vi "Read SEQ.vi"(9 "SEQ file path":path, 10 "Sequence files handle":T1) -> (0 "error out":errorcluster, 1 "AOI List":i16[][](array[numeric]), 2 "# of Frames":i16)   [LabVIEW 2011]
uses:
  Sequence files handle.ctt
  GLIMPSE Globals.vi
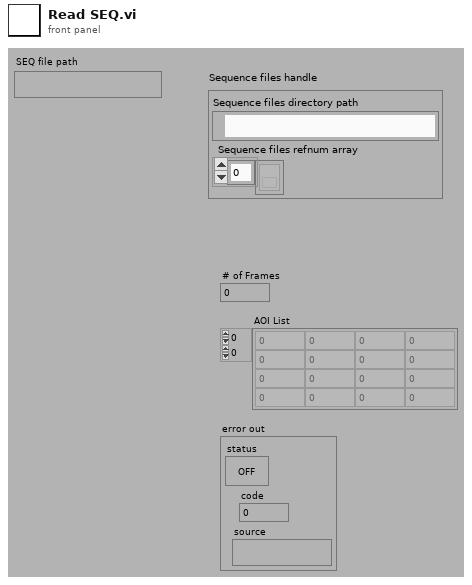
[diagram p1: front panel]
types:
  T1 = typedef "Sequence files handle.ctt" = cluster{"Sequence files directory path":path, "Sequence files refnum array":refnum<file>[]}
  T2 = enum32{"existing file", "new file", "new or existing file", "existing dir", "new dir", "new or existing dir", "existing file (use LLBs)", "new file (use LLBs)", "new or existing file (use LLBs)", "new or existing file or directory (use LLBs)"}
  T3 = cluster{"second":i32, "minute":i32, "hour":i32, "day of month":i32, "month":i32, "year":i32, "day of week":i32, "day of year":i32, "is DST":i32}
  T4 = cluster{"User Name":string, "Description":string, "Time Info":string}
  T5 = typedef "Offset table.ctl" = cluster{"offset":T6, "file number":T7}[]
  T6 = typedef "Offset.ctl" = i32
  T7 = typedef "file number.ctl" = u8
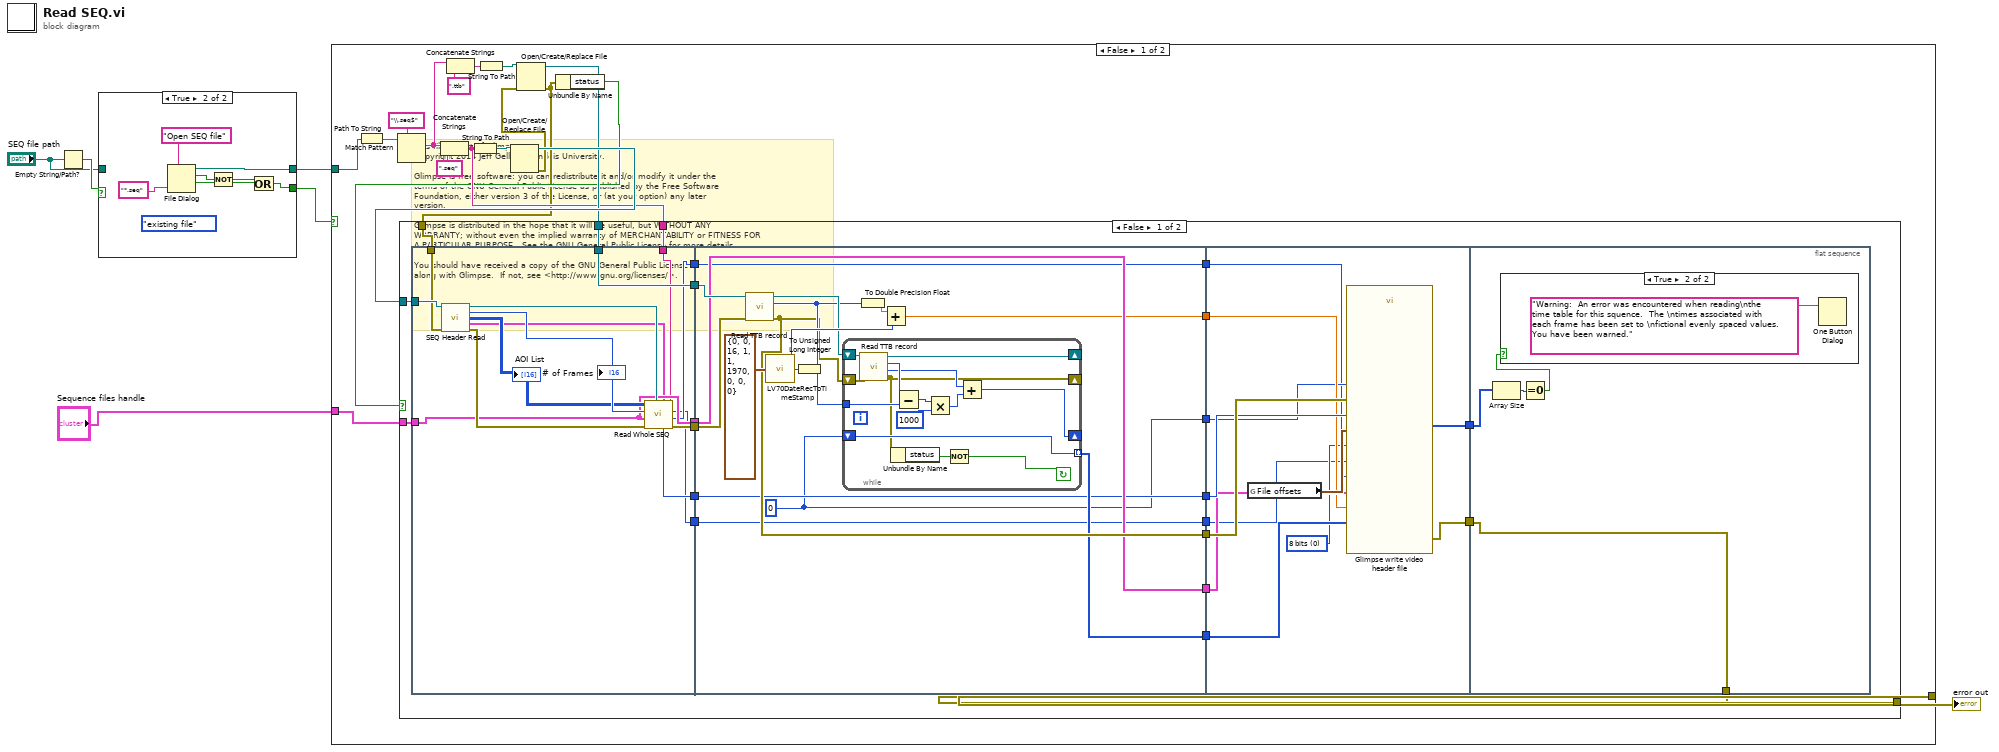
[diagram p0: block diagram]
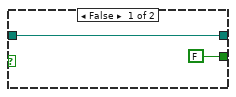
[diagram p2: hidden frame]
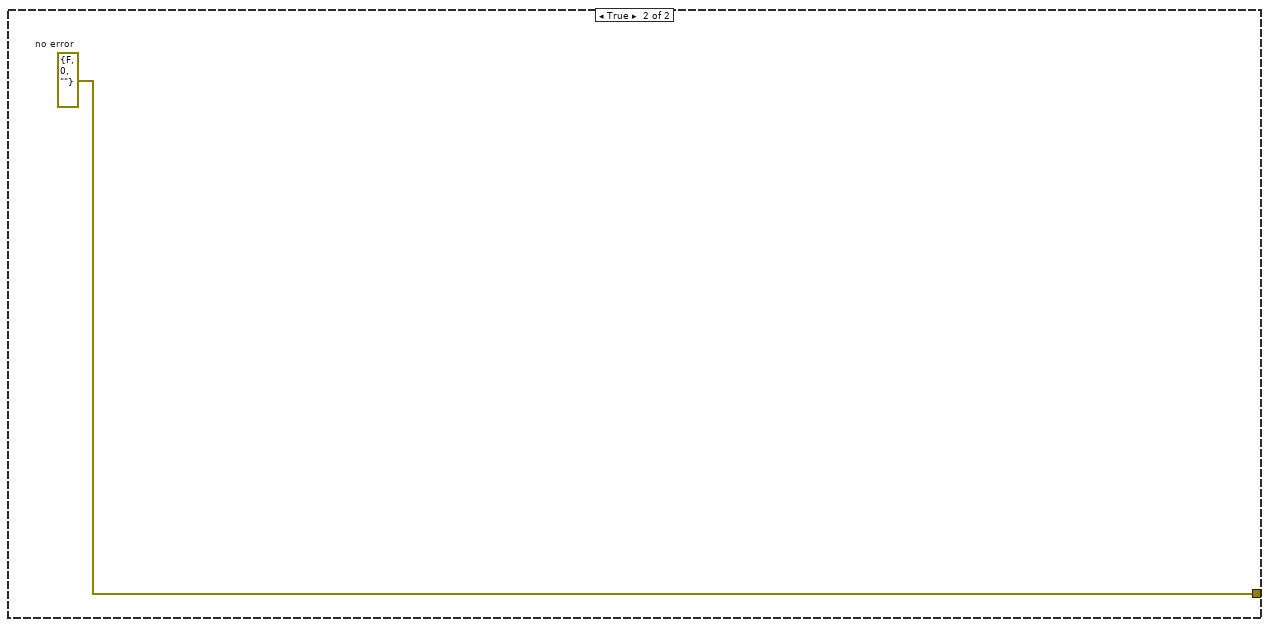
[diagram p5: hidden frame]
diagram:
  # "This file is part of Glimpse. \nCopyright 2014 Jeff Gelles, Brandeis University.    \n\nGlimpse is free software: you can redistribute it and/or modify it under the \nterms of the GNU General Public License as published by the Free Software \nFoundation, either version 3 of the License, or (at your option) any later \nversion.\n\nGlimpse is distributed in the hope that it will be useful, but WITHOUT ANY \nWARRANTY; without even the implied warranty of MERCHANTABILITY or FITNESS FOR \nA PARTICULAR PURPOSE.  See the GNU General Public License for more details.\n\nYou should have received a copy of the GNU General Public License\nalong with Glimpse.  If not, see <http://www.gnu.org/licenses/>."
  n1 = Empty String/Path?(string/path="SEQ file path") -> (empty?=w6:bool)
  n2 = case shown="True" w6 {
    tunnel: [w8 w15] -> w3
    tunnel: "SEQ file path" -> [w8 _]
    tunnel: [FALSE ("cancelled") w11] -> w4
    frame False {
    }
    frame True {
      (unwired) T2."existing file" ("select mode (2)")
      n3 = File Dialog(6:"*.seq" ("pattern"), 7:"Open SEQ file" ("prompt")) -> (1:w12:bool, 2:w14:bool, 3:w15:path)  [unwired: 1 in, 5 out]
      n4 = Not(x=w14) -> (.not. x?=w13:bool)
      n5 = Or(x=w13, y=w12) -> (x .or. y?=w11:bool)
    }
  }
  n6 = case shown="False" w4 {
    tunnel: [w17 w116] -> w2
    tunnel: w3 -> [w30 _]
    tunnel: "Sequence files handle" -> [w16 _]
    frame False {
      n7 = Path To String(path=w30) -> (string=w29:string)
      n8 = Match Pattern(string=w29, regular expression="\\.seq$") -> (before substring=w23:string)  [unwired: 4 out]
      n9 = Concatenate Strings(w23, ".seq") -> (w21:string)
      n10 = Concatenate Strings(w23, ".ttb") -> (w25:string)
      n11 = String To Path(string=w21) -> (path=w28:path)
      n12 = String To Path(string=w25) -> (path=w26:path)
      n13 = Open/Create/Replace File(file path (use dialog)=w28) -> (refnum out=w27:refnum<file>, error out=w20:errorcluster)  [unwired: 1 in, 5 out]
      n14 = Open/Create/Replace File(file path (use dialog)=w26, error in=w20) -> (refnum out=w22:refnum<file>, error out=w18:errorcluster)  [unwired: 5 out]
      n15 = Unbundle By Name(w18) -> ("status"=w19:bool)
      n16 = case shown="False" w19 {
        tunnel: [w50 w115] -> w17
        tunnel: w27 -> [w54 _]
        tunnel: w22 -> [w53 _]
        tunnel: w21 -> [w52 _]
        tunnel: w18 -> [w37 w115]
        tunnel: w16 -> [w51 _]
        frame False {
          n17 = flat-sequence {
            tunnel: w54 -> [w68]
            tunnel: w53 -> [w60]
            tunnel: [w60] -> w49
            tunnel: w52 -> [w59]
            tunnel: w51 -> [w62]
            tunnel: [w62] -> w48
            tunnel: [w63] -> w47
            tunnel: [w61] -> w46
            tunnel: w37 -> [w57]
            tunnel: [w56] -> w35
            tunnel: [w55] -> w33
            tunnel: w49 -> [w84]
            tunnel: w48 -> [w74]
            tunnel: [w74] -> w45
            tunnel: w47 -> [w83]
            tunnel: [w76] -> w44
            tunnel: [w77] -> w43
            tunnel: w46 -> [w73]
            tunnel: [w73] -> w42
            tunnel: [w72] -> w39
            tunnel: [w71] -> w38
            tunnel: [w70] -> w36
            tunnel: w35 -> [w70]
            tunnel: [w69] -> w34
            tunnel: w33 -> [w69]
            tunnel: w45 -> [w104]
            tunnel: [w105] -> w41
            tunnel: w44 -> [w109]
            tunnel: [w109] -> w40
            tunnel: w43 -> [w108]
            tunnel: w42 -> [w106]
            tunnel: w39 -> [w103]
            tunnel: w38 -> [w102]
            tunnel: w36 -> [w100]
            tunnel: w34 -> [w99]
            tunnel: [w110] -> w50
            tunnel: w41 -> [w110]
            tunnel: w40 -> [w112]
            frame #0 {
              n18 = call "SEQ Header Read.vi"("refnum"=w68, "error in"=w57) -> ("refnum out"=w67:refnum<file>, "# of Frames"=w66:i16, "AOI List"=w65:i16[][], "Header Info"=w58:T4, "error out"=w64:errorcluster)  [unwired: 1 in, 8 out]
              "# of Frames" <- w66
              "AOI List" <- w65
              n19 = call "Read Whole SEQ.vi"("AOI List"=w65, "# of Frames"=w66, "Output Sequence files handle"=w62, "error in"=w64, "SEQ file refnum"=w67, "Header Info"=w58, "File name"=w59) -> ("# of frames read"=w61:i32, "Frame height"=w55:i16, "Frame width"=w56:i16, "error out"=w63:errorcluster)
            }
            frame #1 {
              w71 = u32 0 ("Element 0 of TTB")
              n20 = call "Read TTB record.vi"("error in"=w83, "Refnum"=w84) -> ("error out"=w77:errorcluster, "seconds"=w78:u32, "Duplicate Refnum"=w79:refnum<file>)  [unwired: 7 out]
              n21 = call <vilib>:"LV70DateRecToTimeStamp.vi"("date time rec"=T3 {"second"=0, "minute"=0, "hour"=16, "day of month"=1, "month"=1, "year"=1970, "day of week"=0, "day of year"=0, "is DST"=0}) -> ("Time Stamp"=w75:timestamp)
              n22 = To Unsigned Long Integer(number=w75) -> (unsigned 32bit integer=w80:u32)
              n23 = while {
                shift-right: [w96] -> _
                shift-left: w79 -> [w97]
                shift-right: [w87] -> _
                shift-left: w77 -> [w98]
                tunnel: w78 -> [w94]
                shift-right: [w89] -> _
                shift-left: w71 -> [w88]
                tunnel: [w88] -> w76 mode=indexing
                stop <- w85 continue-if-true
                n24 = call "Read TTB record.vi"("error in"=w98, "Refnum"=w97) -> ("error out"=w87:errorcluster, "milliseconds"=w91:u16, "seconds"=w95:u32, "Duplicate Refnum"=w96:refnum<file>)  [unwired: 6 out]
                n25 = Unbundle By Name(w87) -> ("status"=w86:bool)
                n26 = Subtract(x=w95, y=w94) -> (x-y=w93:u32)
                n27 = Multiply(x=w93, y=u32 1000) -> (x*y=w92:u32)
                n28 = Not(x=w86) -> (.not. x?=w85:bool)
                n29 = Add(x=w91, y=w92) -> (x+y=w89:u32)
              }
              n30 = To Double Precision Float(number=w78) -> (double precision float=w81:dbl)
              n31 = Add(x=w81, y=w80) -> (x+y=w72:dbl)
            }
            frame #2 {
              w101 = u32 0 items=["8 bits", "16 bits", "Float", "Complex", "RGB", "HSL"] ("Current sequence pixel depth\n(0=8 bit; 1= 16 bit)")
              n32 = global read "GLIMPSE Globals.vi" "File offsets"() -> (w107:T5)
              n33 = call "Glimpse write video header file.vi"("Number of frames"=w106, "Sequence files handle"=w104, "Pixel depth\n(0=8 bit; 1= 16 bit)"=w101, "error in"=w108, "TTB Array"=w109, "Offsets Array"=w107, "Region width"=w100, "Region height"=w99, "Element 0 of TTB"=w102, "time of 1st frame, \nsec since 1/1/04"=w103) -> ("error out"=w105:errorcluster)  [unwired: 9 in]
            }
            frame #3 {
              n34 = Array Size(array=w112) -> (size(s)=w113:i32)
              n35 = Equal To 0?(x=w113) -> (x = 0?=w111:bool)
              n36 = case shown="True" w111 {
                frame False {
                }
                frame True {
                  n37 = One Button Dialog(message="Warning:  An error was encountered when reading\nthe time table for this squence.  The \ntimes associated with each frame has been set to \nfictional evenly spaced values.  You have been warned.") -> ()  [unwired: 2 out]
                }
              }
            }
          }
        }
        frame True {
        }
      }
    }
    frame True {
      w116 = errorcluster {"status"=FALSE, "code"=0, "source"=""}  # no error
    }
  }
  "error out" <- w2
